vi "RDB Extract Contact_Point Payload.vi"(11 "RDB Message":string) -> (3 "Contact_Point payload":u8[](array[numeric]))   [LabVIEW 2023, in "RDB.lvlib"]
uses:
  RDB.lvlib
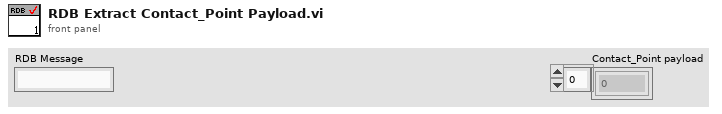
[diagram p1: front panel]
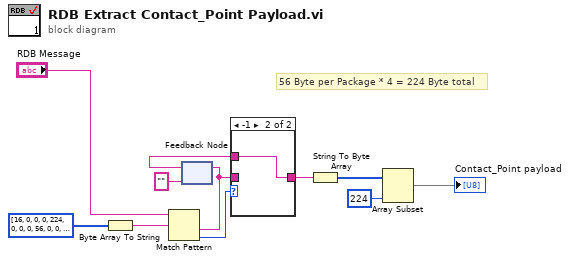
[diagram p0: block diagram]
diagram:
  # "56 Byte per Package * 4 = 224 Byte total"
  n1 = Byte Array To String(unsigned byte array=i32[] [16, 0, 0, 0, 224, 0, 0, 0, 56, 0, 0, 0, 19, 0, 0, 0]) -> (string=w10:string)
  n2 = Match Pattern(string="RDB Message", regular expression=w10) -> (after substring=w4:string, offset past match=w7:i32)  [unwired: 1 in, 2 out]
  n3 = feedback #1("") -> (w3:string)
  n4 = feedback-in #1(w4) -> ()
  n5 = case shown="-1" w7 {
    tunnel: w4 -> [w12 _]
    tunnel: [w12 w13] -> w6
    tunnel: w3 -> [_ w13]
    frame 0, Default {
    }
    frame -1 {
    }
  }
  n6 = String To Byte Array(string=w6) -> (unsigned byte array=w9:u8[])
  n7 = Array Subset(array=w9, length=224) -> (→"Contact_Point payload":u8[])  [unwired: 1 in]
